vi "test Acyclic Loopback.vi"(8 "error in":errorcluster, 11 "TestCase in":refnum<class "Octal Loopback.lvclass">) -> (0 "error out":errorcluster, 3 "TestCase out":refnum<class "Octal Loopback.lvclass">)   [LabVIEW 2020, in "Octal Loopback.lvclass"]
uses:
  Octal Loopback.lvclass
  C:/Program Files (x86)/National Instruments/LabVIEW 2020/vi.lib/NI/VeriStand Custom Device Testing Tools/VeriStandTestCase/VeriStandTestCase.lvclass
  <vilib>/numeric/Random Number (Range) U64.vi
  <vilib>/numeric/sub_Random U32.vi
  <vilib>/NI VeriStand/Execution/Workspace/NI VeriStand - Set Multiple Channel Values.vi
  <vilib>/addons/_JKI Toolkits/VI Tester/TestCase.llb/TestCase.lvclass
  <vilib>/NI VeriStand/Execution/Workspace/NI_VS Workspace ExecutionAPI.lvlib
  <vilib>/NI/VeriStand Custom Device Testing Tools/VeriStandTestUtilities/VeriStandTestUtilities.lvlib
  C:/Program Files (x86)/National Instruments/LabVIEW 2020/vi.lib/addons/_JKI Toolkits/VI Tester/TestCase.llb/TestCase.lvclass
  C:/Users/nitest/Desktop/Git 2020/niveristand-ballard-arinc429-custom-device/Source/Custom Device Support/Tests/System/Octal Loopback/Octal Loopback.lvclass
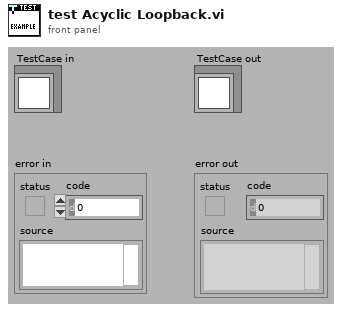
[diagram p1: front panel]
types:
  T1 = typedef "NI_VS Workspace ExecutionAPI.lvlib/WorkspaceAPI.ctl" = refnum<k24>
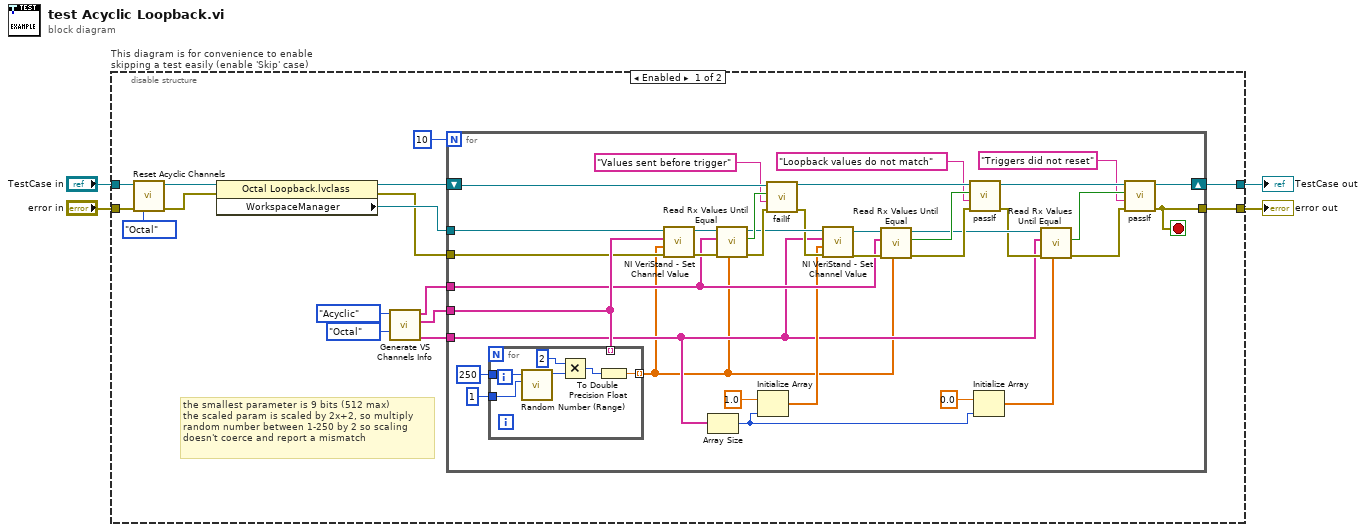
[diagram p0: block diagram]
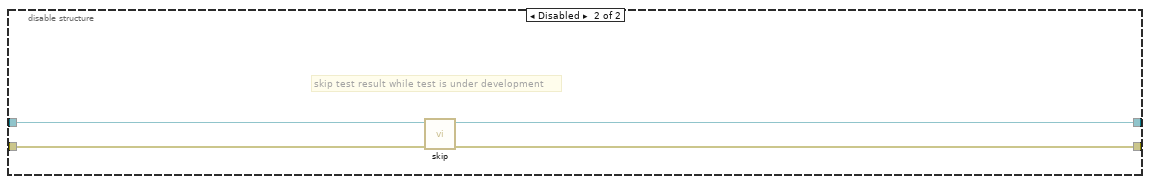
[diagram p2: hidden frame]
diagram:
  n1 = disable-structure "This diagram is for convenience to enable skipping a test easily (enable 'Skip' case)" shown="Enabled" {
    disable-tunnel: "TestCase in" -> [w8 w65]
    disable-tunnel: [w14 w63] -> w1
    disable-tunnel: [w13 w64] -> w3
    disable-tunnel: "error in" -> [w15 w62]
    frame Enabled {
      # "the smallest parameter is 9 bits (512 max)\nthe scaled param is scaled by 2x+2, so multiply \nrandom number between 1-250 by 2 so scaling\ndoesn't coerce and report a mismatch"
      n2 = call "Reset Acyclic Channels.vi"("error in (no error)"=w15, "Label Format (Decimal)"=enum16{"Decimal", "Octal"}."Octal", "reference in"=w8) -> ("error out"=w9:errorcluster, "reference out"=w7:refnum<class "Octal Loopback.lvclass">)  [unwired: 7 in]
      n3 = property class="Octal Loopback.lvclass"(reference=w7, error in=w9) -> (reference out=w17:refnum<class "Octal Loopback.lvclass">, error out=w18:errorcluster, "WorkspaceManager"=w19:T1)
      n4 = call "Generate VS Channels Info.vi"("Label Format (Decimal)"=enum16{"Decimal", "Octal"}."Octal", "Transfer Type"=enum16{"Acyclic", "Scheduled"}."Acyclic") -> ("Tx Trigger Channels Array"=w11:string[], "Tx Channels Array"=w12:string[], "Rx Channels Array"=w20:string[])  [unwired: 5 in, 2 out]
      n5 = for {
        N: 10 -> [_]
        tunnel: w20 -> [w41]
        tunnel: w19 -> [w53]
        tunnel: w18 -> [w46]
        tunnel: w12 -> [w52]
        shift-right: [w35] -> w14
        shift-left: w17 -> [w48]
        tunnel: [w37] -> w13
        tunnel: w11 -> [w25]
        stop <- w37 stop-if-true
        n6 = for {
          tunnel: [w60] -> w21 mode=indexing
          tunnel: u64 250 ("upper bound (100)") -> [w59]
          tunnel: u64 1 ("upper bound (100)") -> [w58]
          tunnel: w52 -> [_] mode=indexing
          n7 = call-poly <vilib>:"Random Number (Range).vi"("lower bound (0)"=w58, "upper bound (100)"=w59) -> ("number"=w61:u64)  [unwired: 9 in]
          n8 = Multiply(x=u64 2, y=w61) -> (x*y=w57:u64)
          n9 = To Double Precision Float(number=w57) -> (double precision float=w60:dbl)
        }
        n10 = call-poly <vilib>:"NI VeriStand - Set Channel Value.vi"("error in (no error)"=w46, "Values"=w21, "Channels"=w52, "WorkspaceManager in"=w53) -> ("error out"=w49:errorcluster, "WorkspaceManager out"=w51:T1)  [unwired: 6 in]
        n11 = Array Size(array=w25) -> (size(s)=w22:i32)
        n12 = call <vilib>:"Read Rx Values Until Equal.vi"("expected values"=w21, "error in"=w49, "Rx aliases"=w41, "workspace manager in"=w51) -> ("error out"=w50:errorcluster, "values equal expected"=w47:bool, "workspace manager out"=w45:T1)  [unwired: 5 in]
        n13 = Initialize Array(1.0, w22) -> (w26:dbl[])
        n14 = call-dynamic "failIf.vi"("error in (no error)"=w50, "message (\"\")"="Values sent before trigger" ("message (\"\")"), "fail"=w47, "TestCase in"=w48) -> ("error out"=w44:errorcluster, "TestCase out"=w38:refnum<class "Octal Loopback.lvclass">)  [unwired: 6 in]
        n15 = call-poly <vilib>:"NI VeriStand - Set Channel Value.vi"("error in (no error)"=w44, "Values"=w26, "Channels"=w25, "WorkspaceManager in"=w45) -> ("error out"=w42:errorcluster, "WorkspaceManager out"=w43:T1)  [unwired: 6 in]
        n16 = call <vilib>:"Read Rx Values Until Equal.vi"("expected values"=w21, "error in"=w42, "Rx aliases"=w41, "workspace manager in"=w43) -> ("error out"=w39:errorcluster, "values equal expected"=w40:bool, "workspace manager out"=w33:T1)  [unwired: 5 in]
        n17 = call-dynamic "passIf.vi"("error in (no error)"=w39, "message (\"\")"="Loopback values do not match" ("message (\"\")"), "pass"=w40, "TestCase in"=w38) -> ("error out"=w32:errorcluster, "TestCase out"=w36:refnum<class "Octal Loopback.lvclass">)  [unwired: 6 in]
        n18 = Initialize Array(0.0, w22) -> (w23:dbl[])
        n19 = call <vilib>:"Read Rx Values Until Equal.vi"("expected values"=w23, "error in"=w32, "Rx aliases"=w25, "workspace manager in"=w33) -> ("error out"=w31:errorcluster, "values equal expected"=w34:bool)  [unwired: 5 in, 1 out]
        n20 = call-dynamic "passIf.vi"("error in (no error)"=w31, "message (\"\")"="Triggers did not reset" ("message (\"\")"), "pass"=w34, "TestCase in"=w36) -> ("error out"=w37:errorcluster, "TestCase out"=w35:refnum<class "Octal Loopback.lvclass">)  [unwired: 6 in]
      }
    }
    frame Disabled {
      # "skip test result while test is under development"
      n21 = call <vilib>:"skip.vi"("error in (no error)"=w62, "TestCase in"=w65) -> ("error out"=w64:errorcluster, "TestCase out"=w63:refnum<class "Octal Loopback.lvclass">)  [unwired: 8 in]
    }
  }
  "error out" <- w3
  "TestCase out" <- w1
